vi "Configure PRACH Modulation EVM Window Length.vi"(8 "error in (no error)":errorcluster, 9 "Modulation EVM Window Length":i32[](array[numeric]), 10 "Instance (1)":T1=1, 11 "VISA resource name":refnum<visa-resource-name>) -> (0 "error out":errorcluster, 3 "VISA resource name out":refnum<visa-resource-name>)   [LabVIEW 2020, in "Rohde&Schwarz CMWXP NR FR1 Measurement.lvlib"]
doc: "Specifies the EVM window length in samples for all preamble formats.\n\nAttribute:\nRSCMWXPNRFR1M_ATTR_PRACH_MODULATION_EVM_WINDOW_LENGTH\n\nRemote-control command:\nCONFigure:NRSub:MEAS<i>:PRACh:MODulation:EWLength"
uses:
  <instrlib>/Rohde&Schwarz CMWXP NR FR1 Measurement/Rohde&Schwarz CMWXP NR FR1 Measurement.lvlib
  <instrlib>/Rohde&Schwarz CMWXP NR FR1 Measurement/Private/_Instance.ctl
  <instrlib>/Rohde&Schwarz CMWXP NR FR1 Measurement/Private/rsidr_core.llb/rsidr_core.lvlib
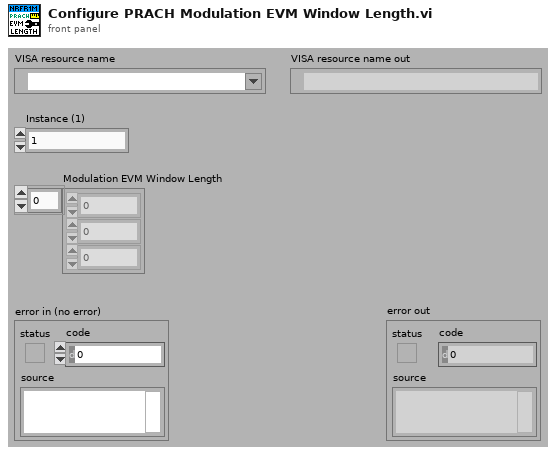
[diagram p1: front panel]
types:
  T1 = typedef "Rohde&Schwarz CMWXP NR FR1 Measurement.lvlib/_Instance.ctl" = i32
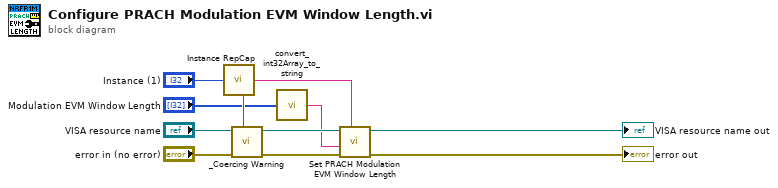
[diagram p0: block diagram]
diagram:
  n1 = call <instrlib>:"Instance RepCap.vi"("Instance In"="Instance (1)") -> ("In Range?"=w4:bool, "RepCap Identifier Out"=w3:string)  [unwired: 1 in]
  n2 = call <instrlib>:"_Coercing Warning.vi"("In Range?"=w4, "error in (no error)"="error in (no error)", "VISA resource name"="VISA resource name") -> ("error out"=w7:errorcluster, "VISA resource name out"=w6:refnum<visa-resource-name>)  [unwired: 7 in]
  n3 = call <instrlib>:"convert_int32Array_to_string.vi"("I32 array in"="Modulation EVM Window Length") -> ("string out"=w1:string)  [unwired: 4 in]
  n4 = call "Set PRACH Modulation EVM Window Length"("Repeated Capabilities"=w3, "error in (no error)"=w7, "PRACH Modulation EVM Window Length ()"=w1, "instrument handle"=w6) -> ("error out"=→"error out":errorcluster, "instrument handle out"=→"VISA resource name out":refnum<visa-resource-name>)  [unwired: 6 in]
